vi "Reset.vi"(8 "error in (no error)":errorcluster, 11 "ChromaPowerSupply in":refnum<class "ChromaPowerSupply.lvclass">) -> (0 "error out":errorcluster, 3 "ChromaPowerSupply out":refnum<class "ChromaPowerSupply.lvclass">)   [LabVIEW 2018, in "AcPwrPlugins.lvlib" / "ChromaPowerSupply.lvclass"]
doc: "This VI resets the instrument(s) into a know state."
uses:
  ChromaPowerSupply.lvclass
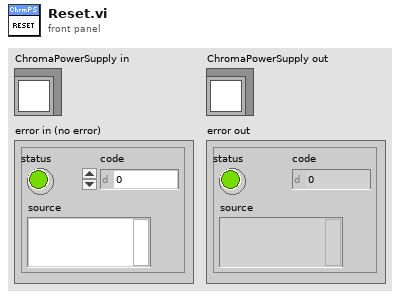
[diagram p1: front panel]
types:
  T1 = typedef "AcPwrPlugins.lvlib/ChromaPowerSupply.lvclass/Measurements.ctl" = cluster{"Handle":string, "Name":string, "Enabled":bool, "Measurement Value":dbl, "btnMeasFetch":bool, "ProtectionStatusString":string, "Measurement Type":enum16{"Voltage", "Current", "Power"}}[]
  T2 = typedef "AcPwrPlugins.lvlib/ChromaPowerSupply.lvclass/Device(s)Settings.ctl" = cluster{"Phases":cluster{"Handle":string, "Instrument Options":string, "id query (T)":bool, "reset device (T)":bool, "Timing":cluster{"TimingOn":enum16{""}, "Hours":u32, "Minutes":u32, "Seconds":dbl, "CutoffVoltage":dbl}, "Connected":bool, "Output Mode":enum16{"Voltage (DC)", "Current (DC)"}, "Voltage":dbl, "Current":dbl, "High Voltage Limit":dbl, "High Current Limit":dbl, "Power Protect":dbl, "Current Protect":dbl, "Voltage Protect":dbl, "Low Current Limit":dbl, "Low Voltage Limit":dbl, "Current Slew Rate":dbl, "Voltage Slew Rate":dbl, "Current Slew Infinite?":bool}[], "MeasName":string}
  T3 = cluster{"Handle":string, "Instrument Options":string, "id query (T)":bool, "reset device (T)":bool, "Timing":cluster{"TimingOn":enum16{""}, "Hours":u32, "Minutes":u32, "Seconds":dbl, "CutoffVoltage":dbl}, "Connected":bool, "Output Mode":enum16{"Voltage (DC)", "Current (DC)"}, "Voltage":dbl, "Current":dbl, "High Voltage Limit":dbl, "High Current Limit":dbl, "Power Protect":dbl, "Current Protect":dbl, "Voltage Protect":dbl, "Low Current Limit":dbl, "Low Voltage Limit":dbl, "Current Slew Rate":dbl, "Voltage Slew Rate":dbl, "Current Slew Infinite?":bool}[]
  T4 = cluster{"Handle":string, "Instrument Options":string, "id query (T)":bool, "reset device (T)":bool, "Timing":cluster{"TimingOn":enum16{""}, "Hours":u32, "Minutes":u32, "Seconds":dbl, "CutoffVoltage":dbl}, "Connected":bool, "Output Mode":enum16{"Voltage (DC)", "Current (DC)"}, "Voltage":dbl, "Current":dbl, "High Voltage Limit":dbl, "High Current Limit":dbl, "Power Protect":dbl, "Current Protect":dbl, "Voltage Protect":dbl, "Low Current Limit":dbl, "Low Voltage Limit":dbl, "Current Slew Rate":dbl, "Voltage Slew Rate":dbl, "Current Slew Infinite?":bool}
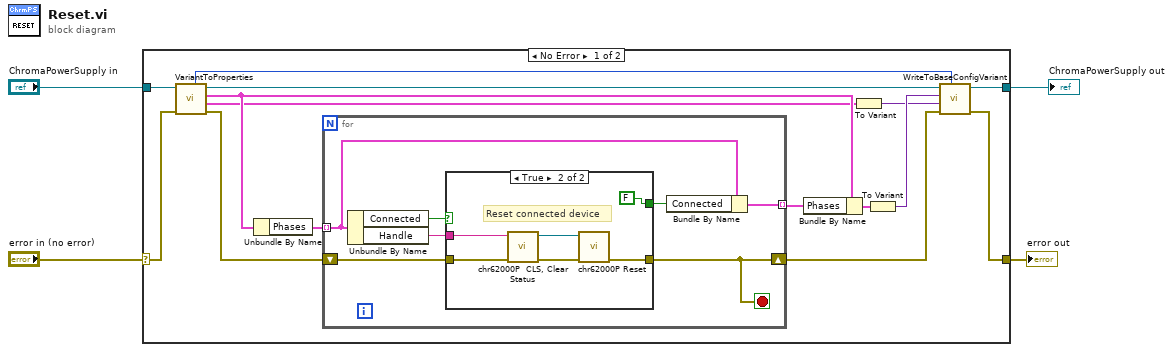
[diagram p0: block diagram]
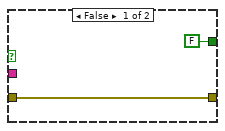
[diagram p2: hidden frame]
diagram:
  n1 = case shown="No Error" "error in (no error)" {
    selector: "error in (no error)" -> [w18 w36]
    tunnel: [w10 w36] -> w1
    tunnel: [w12 w35] -> w2
    tunnel: "ChromaPowerSupply in" -> [w19 w35]
    frame No Error {
      n2 = call-dynamic "VariantToProperties.vi"("error in (no error)"=w18, "ChromaPowerSupply in"=w19) -> ("error out"=w17:errorcluster, "Measurements"=w8:T1, "Device Settings"=w14:T2, "ChromaPowerSupply out"=w15:refnum<class "ChromaPowerSupply.lvclass">, "Measurement Refresh Time (ms)"=w5:u32)  [unwired: 5 in]
      n3 = Unbundle By Name(w14) -> ("Phases"=w16:T3)
      n4 = for {
        tunnel: w16 -> [w22] mode=indexing
        shift-right: [w24] -> w11
        shift-left: w17 -> [w26]
        tunnel: [w20] -> w13 mode=indexing
        stop <- w24 stop-if-true
        n5 = Unbundle By Name(w22) -> ("Connected"=w23:bool, "Handle"=w25:string)
        n6 = case shown="True" w23 {
          tunnel: w26 -> [w28 w31]
          tunnel: w25 -> [_ w32]
          tunnel: [w28 w34] -> w24
          tunnel: [FALSE FALSE] -> w21
          frame False {
          }
          frame True {
            # "Reset connected device"
            n7 = call <instrlib>:"chr62000P  CLS, Clear Status.vi"("error in (no error)"=w31, "instrument handle"=w32) -> ("error out"=w30:errorcluster, "instrument handle out"=w29:refnum<k15>)  [unwired: 8 in]
            n8 = call <instrlib>:"chr62000P Reset.vi"("error in (no error)"=w30, "instrument handle"=w29) -> ("error out"=w34:errorcluster)  [unwired: 8 in, 1 out]
          }
        }
        n9 = Bundle By Name(cluster=w22, "Connected"=w21) -> (w20:T4)
      }
      n10 = Bundle By Name(cluster=w14, "Phases"=w13) -> (w9:T2)
      n11 = To Variant(anything=w8) -> (Variant=w6:variant)
      n12 = To Variant(anything=w9) -> (Variant=w7:variant)
      n13 = call-dynamic "WriteToBaseConfigVariant.vi"("Measurement Refresh Time (ms)"=w5, "error in (no error)"=w11, "Meas"=w6, "Config"=w7, "ChromaPowerSupply in"=w15) -> ("error out"=w10:errorcluster, "ChromaPowerSupply out"=w12:refnum<class "ChromaPowerSupply.lvclass">)  [unwired: 5 in]
    }
    frame Error {
    }
  }
  "error out" <- w1
  "ChromaPowerSupply out" <- w2
